vi "MagX Probe List.vi"(2 "Probe  list":i32(listbox)=-1, 6 "Days range":dbl=90.0, 8 "error in":errorcluster, 9 "Current station in":string, 10 "Initial Selection":string, 11 "Hub URL":string="magfair.lanl.gov") -> (0 "error out":errorcluster, 1 "OK":bool, 3 "Probe info":T1={"instrumentPid"="Undocumented", "title"="", "filename"="", "filestorePath"="", "createDate"="", "modifyDate"="", "categories"="", "instrumenType"=""})   [LabVIEW 2025]
uses:
  Instrument info.ctl
  Experiment info.ctl
panel:
  out "Current probe":string
  out "Selection":string
  in  "Select":bool
  out "Probes":T1[](array[typedef])
  out "resulting string":string
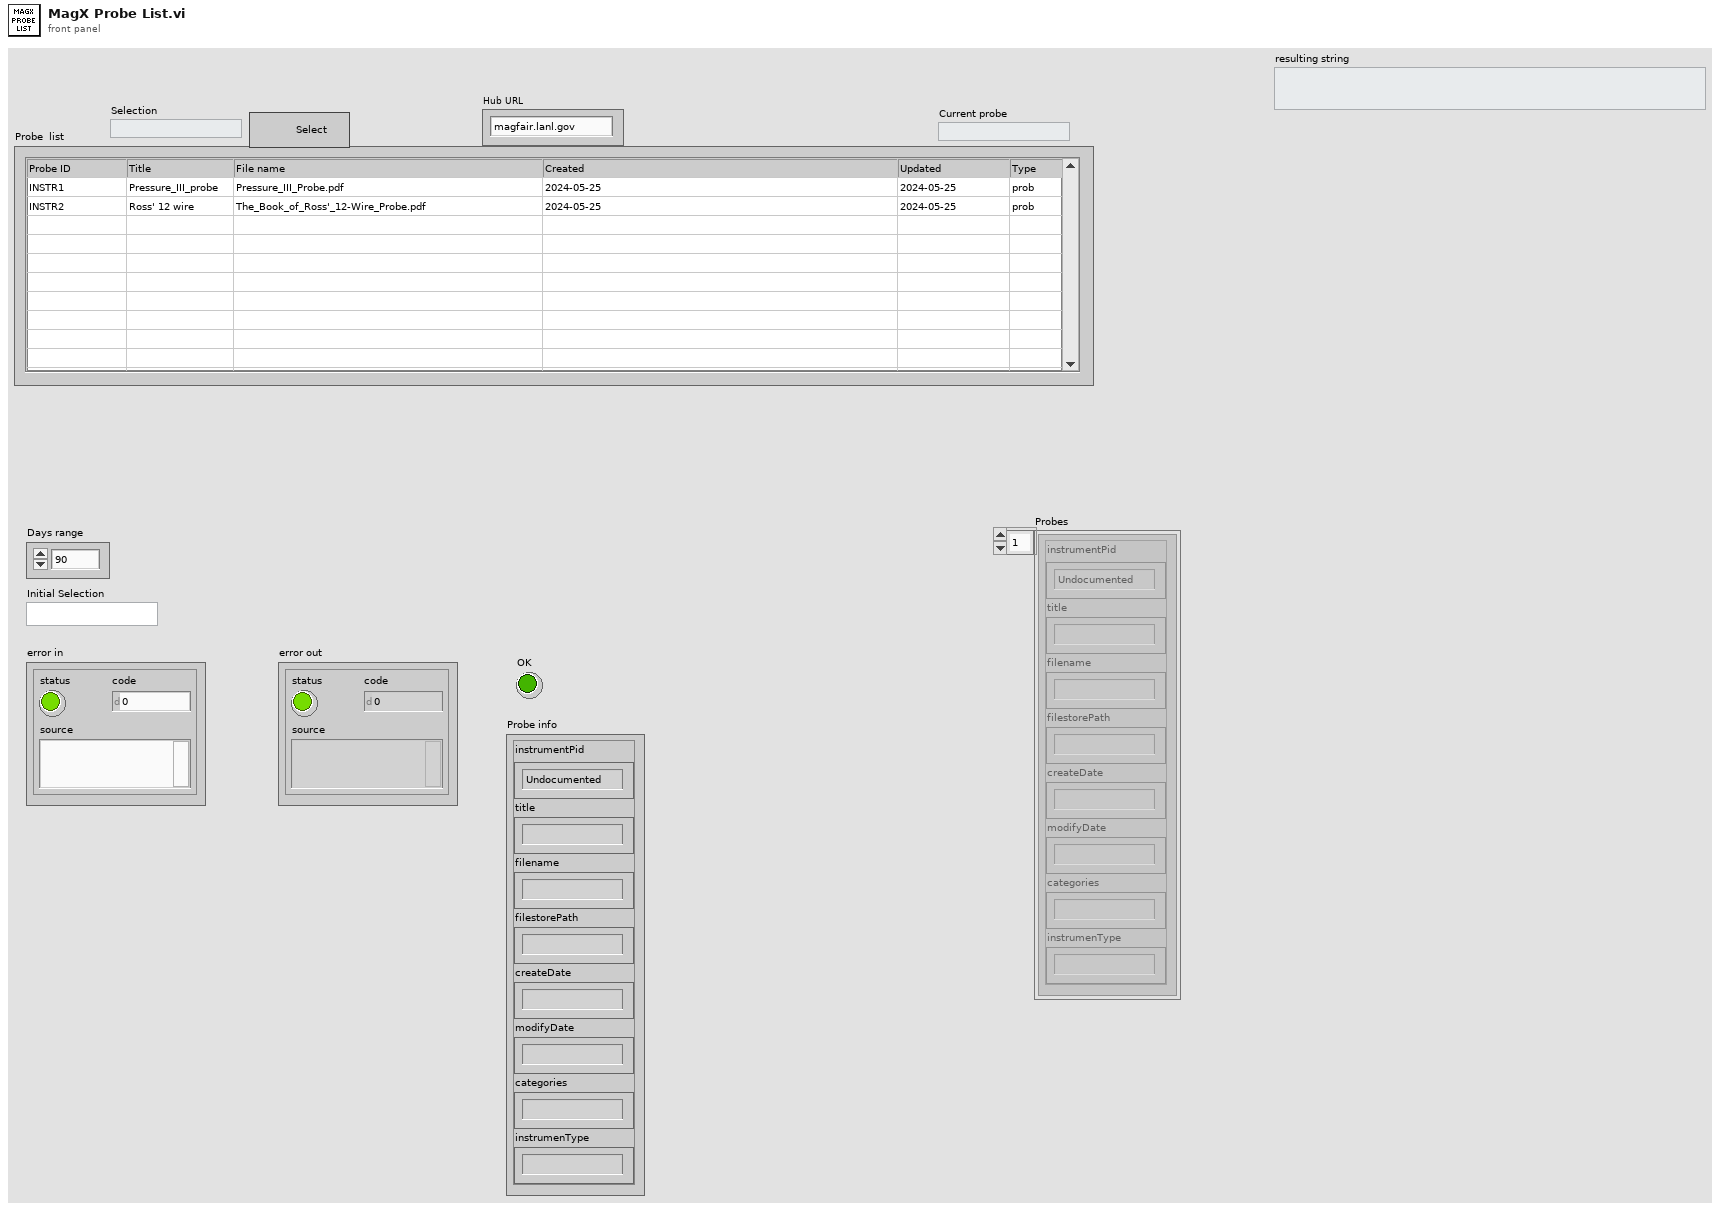
[diagram p1: front panel]
types:
  T1 = typedef "Instrument info.ctl" = cluster{"instrumentPid":string, "title":string, "filename":string, "filestorePath":string, "createDate":string, "modifyDate":string, "categories":string, "instrumenType":string}
  T2 = typedef "Experiment info.ctl" = cluster{"attendee":string[], "title":string, "magnet_System":string, "proposal_Number":string, "proposal_Title":string, "facility":string, "pi":string, "dtstart":string, "dtend":string, "dtstamp":string, "location":string, "summary":string, "pid":string, "support":string, "uid":string, "start":u64, "id":u64}
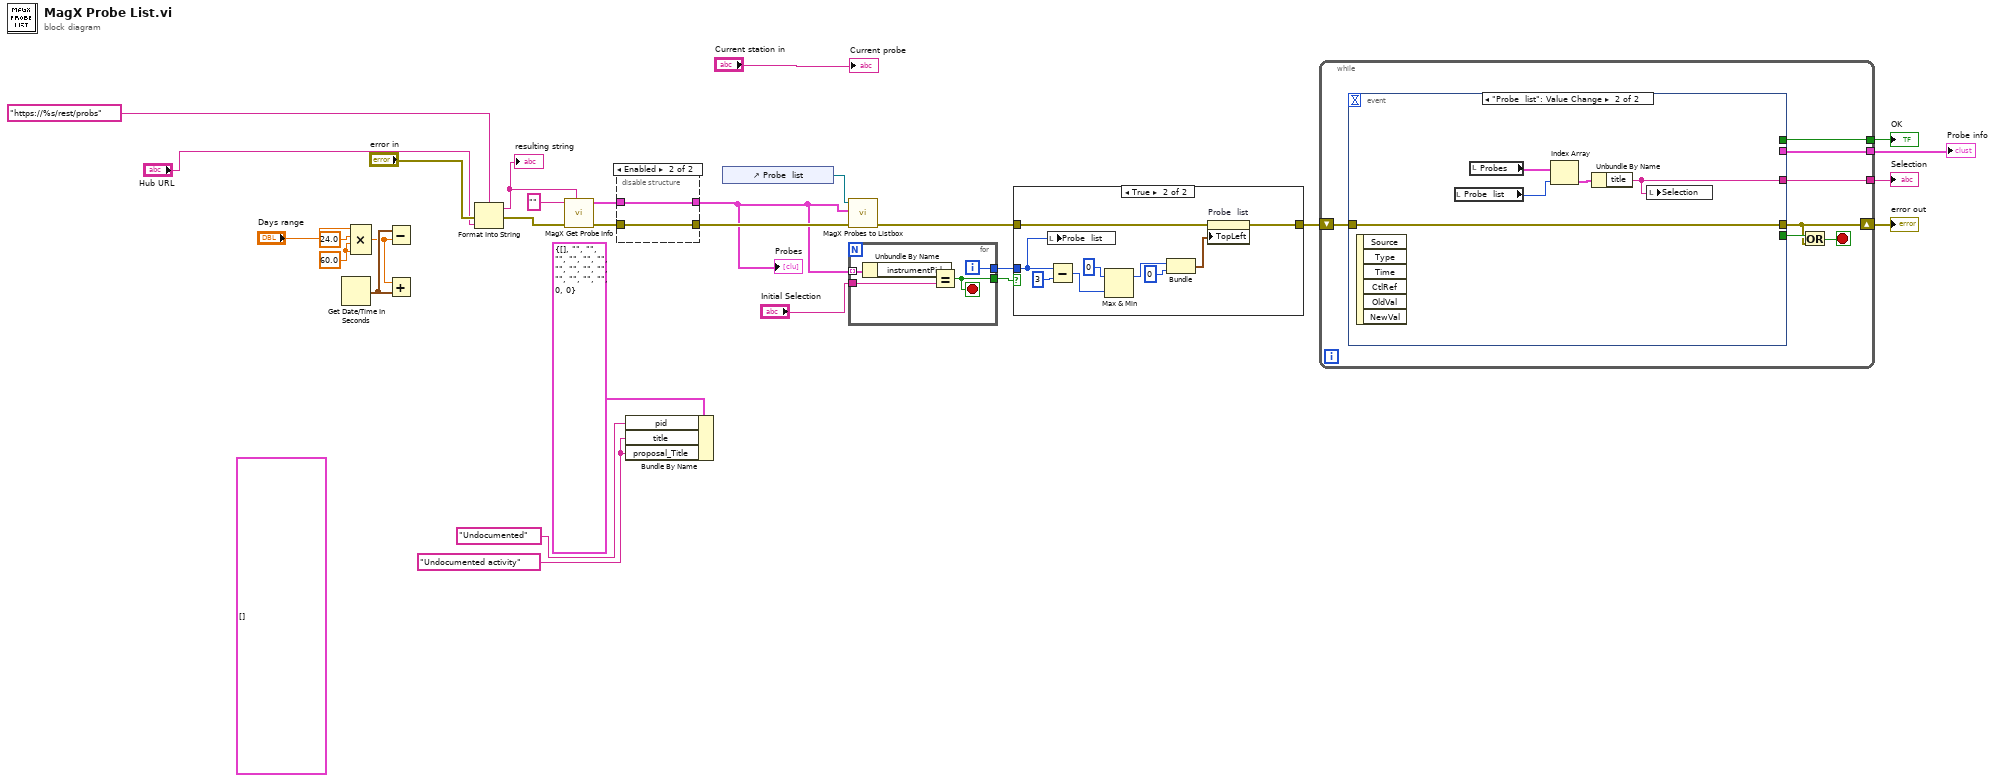
[diagram p0: block diagram]
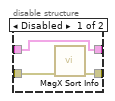
[diagram p2: hidden frame]
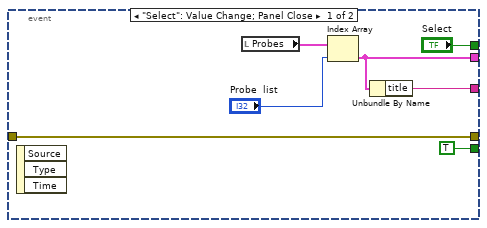
[diagram p4: hidden frame]
diagram:
  (unwired) T2[] [] ("Data in 2")
  w9 = "Undocumented activity"
  w28 = 60.0
  n1 = Get Date/Time In Seconds() -> (seconds since 1Jan1904=w27:timestamp)
  n2 = Compound Arithmetic op=MULTIPLY("Days range", 24.0, w28, w28) -> (w25:dbl)
  n3 = Subtract(x=w27, y=w25) -> ()  [unwired: 1 out]
  n4 = Add(x=w25, y=w27) -> ()  [unwired: 1 out]
  n5 = Format Into String(format string="https://%s/rest/probs", error in="error in", "Hub URL") -> (resulting string=w23:string, error out=w21:errorcluster)  [unwired: 1 in]
  "resulting string" <- w23
  n6 = call "MagX Get Probe Info.vi"("url"=w23, "error in"=w21, "Station"="") -> ("error out"=w6:errorcluster, "Data out"=w4:T1[])  [unwired: 7 in]
  n7 = disable-structure shown="Enabled" {
    disable-tunnel: w6 -> [w32 w33]
    disable-tunnel: [w31 w33] -> w5
    disable-tunnel: w4 -> [w30 w34]
    disable-tunnel: [w30 w34] -> w3
    frame Disabled {
      n8 = call "MagX Sort Info.vi"("error in"=w32) -> ("error out"=w31:errorcluster)  [unwired: 9 in, 1 out]
    }
    frame Enabled {
    }
  }
  "Probes" <- w3
  n9 = Bundle By Name(cluster=T2 {"attendee"=[], "title"="", "magnet_System"="", "proposal_Number"="", "proposal_Title"="", "facility"="", "pi"="", "dtstart"="", "dtend"="", "dtstamp"="", "location"="", "summary"="", "pid"="", "support"="", "uid"="", "start"=0, "id"=0} ("Experiment info"), "pid"="Undocumented", "title"=w9, "proposal_Title"=w9) -> ()  [unwired: 1 out]
  n10 = control-ref of="Probe  list"() -> (w20:refnum<vi>)
  n11 = call "MagX Probes to Listbox.vi"("error in"=w5, "Probes"=w3, "Listbox ref"=w20) -> ("error out"=w13:errorcluster)  [unwired: 7 in, 1 out]
  n12 = for {
    tunnel: w3 -> [w39] mode=indexing
    tunnel: "Initial Selection" -> [w38]
    tunnel: [w36] -> w14
    tunnel: [w35] -> w15
    i -> [w36]
    stop <- w35 stop-if-true
    n13 = Unbundle By Name(w39) -> ("instrumentPid"=w37:string)
    n14 = Equal?(x=w37, y=w38) -> (x = y?=w35:bool)
  }
  n15 = case shown="True" w15 {
    tunnel: w14 -> [_ w49]
    tunnel: w13 -> [w40 w45]
    tunnel: [w40 w44] -> w12
    frame False {
    }
    frame True {
      n16 = local write "Probe  list"(w49) -> ()
      n17 = Subtract(x=w49, y=3) -> (x-y=w42:i32)
      n18 = Max & Min(x=0, y=w42) -> (max(x,y)=w43:i32)  [unwired: 1 out]
      n19 = Bundle(w43, 0) -> (w48:cluster{i32, i32})  [unwired: 1 in]
      n20 = property on="Probe  list" class="MCListbox (strict)"(error in=w45, "TopLeft"=w48) -> (error out=w44:errorcluster)  [unwired: 1 in, 1 out]
    }
  }
  n21 = while {
    shift-right: [w53] -> w17
    shift-left: w12 -> [w56]
    tunnel: [w52] -> w18
    tunnel: [w51] -> w8
    tunnel: [w50] -> w7
    stop <- w54 stop-if-true
    n22 = event shown="[1] \"Probe  list\": Value Change" {
      selector: _ -> [_ _]
      dyn-events: _ -> [_ _]
      timeout: _ -> [_ _]
      tunnel: w56 -> [w63 w68]
      tunnel: [w63 w68] -> w53
      tunnel: [TRUE ("Select") _] -> w55
      tunnel: [w60 w64] -> w52
      tunnel: [w58 _] -> w51
      tunnel: ["Select" _] -> w50
      event "Select": Value Change; Panel Close {
        n23 = event-data() -> ()  [unwired: 1 in, 3 out]
        n24 = local read "Probes"() -> (w62:T1[])
        n25 = Index Array(array=w62, index="Probe  list") -> (element=w58:T1)
        n26 = Unbundle By Name(w58) -> ("title"=w60:string)
      }
      event "Probe  list": Value Change {
        n27 = event-data() -> ()  [unwired: 1 in, 6 out]
        n28 = local read "Probe  list"() -> (w65:i32)
        n29 = local read "Probes"() -> (w67:T1[])
        n30 = Index Array(array=w67, index=w65) -> (element=w66:T1)
        n31 = Unbundle By Name(w66) -> ("title"=w64:string)
        n32 = local write "Selection"(w64) -> ()
      }
    }
    n33 = Or(x=w55, y=w53) -> (x .or. y?=w54:bool)
  }
  "error out" <- w17
  "Selection" <- w18
  "Probe info" <- w8
  "OK" <- w7
  "Current probe" <- "Current station in"
